vi "Sorted Data Demo.vi"() -> ()   [LabVIEW 2011]
uses:
  Ordered Array/Ordered Array.lvclass
panel:
  out "Combined Array":u32[](array[numeric])
  out "Array 2":u32[](array[numeric])
  out "Array 1":u32[](array[numeric])
  # "The Ordered Array class represents an array, but it is an array that guarantees that its elements are in order. The encapsulation ensures that no element can be added to the array except by going through the class' interface, and that interface guarantees the array remains sorted."
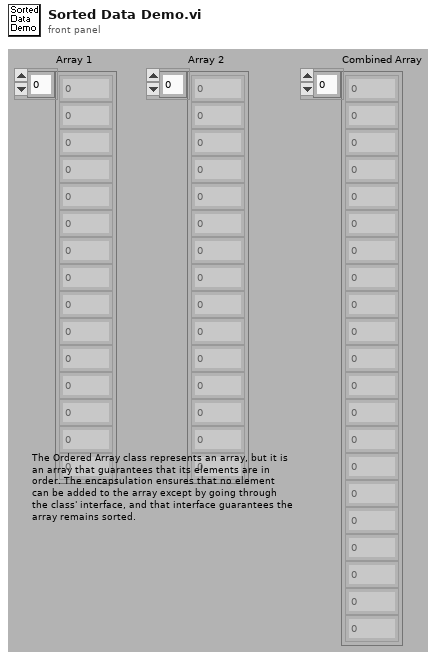
[diagram p1: front panel]
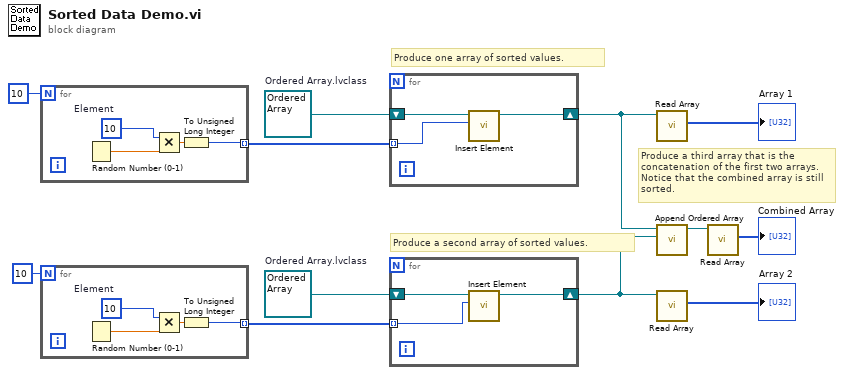
[diagram p0: block diagram]
diagram:
  w7 = refnum<class "Ordered Array.lvclass"> refnum  # Ordered Array.lvclass
  w12 = refnum<class "Ordered Array.lvclass"> refnum  # Ordered Array.lvclass
  # "Produce a third array that is the \nconcatenation of the first two arrays. Notice that the combined array is still sorted."
  # "Produce a second array of sorted values."
  # "Produce one array of sorted values."
  n1 = for {
    N: 10 -> [_]
    tunnel: [w13] -> w9 mode=indexing
    w16 = u32 10  # Element
    n2 = Random Number (0-1)() -> (number: 0 to 1=w15:dbl)
    n3 = Multiply(x=w16, y=w15) -> (x*y=w14:dbl)
    n4 = To Unsigned Long Integer(number=w14) -> (unsigned 32bit integer=w13:u32)
  }
  n5 = for {
    N: 10 -> [_]
    tunnel: [w17] -> w1 mode=indexing
    w20 = u32 10  # Element
    n6 = Random Number (0-1)() -> (number: 0 to 1=w19:dbl)
    n7 = Multiply(x=w20, y=w19) -> (x*y=w18:dbl)
    n8 = To Unsigned Long Integer(number=w18) -> (unsigned 32bit integer=w17:u32)
  }
  n9 = for {
    shift-right: [w22] -> w6
    shift-left: w12 -> [w23]
    tunnel: w9 -> [w21] mode=indexing
    n10 = call "Insert Element.vi"("Element"=w21, "Ordered Array in"=w23) -> ("Ordered Array out"=w22:refnum<class "Ordered Array.lvclass">)  [unwired: 8 in, 1 out]
  }
  n11 = for {
    shift-right: [w25] -> w5
    shift-left: w7 -> [w26]
    tunnel: w1 -> [w24] mode=indexing
    n12 = call "Insert Element.vi"("Element"=w24, "Ordered Array in"=w26) -> ("Ordered Array out"=w25:refnum<class "Ordered Array.lvclass">)  [unwired: 8 in, 1 out]
  }
  n13 = call "Read Array.vi"("Ordered Array.lvclass in"=w6) -> ("Array"=→"Array 1":u32[])  [unwired: 9 in, 1 out]
  n14 = call "Append Ordered Array.vi"("Ordered Array 2 in"=w5, "Ordered Array in"=w6) -> ("Ordered Array out"=w3:refnum<class "Ordered Array.lvclass">)  [unwired: 8 in, 1 out]
  n15 = call "Read Array.vi"("Ordered Array.lvclass in"=w5) -> ("Array"=→"Array 2":u32[])  [unwired: 9 in, 1 out]
  n16 = call "Read Array.vi"("Ordered Array.lvclass in"=w3) -> ("Array"=→"Combined Array":u32[])  [unwired: 9 in, 1 out]
